vi "Create Plot Object.vi"(6 "Control Ref Queue":T1, 7 "Actual Transform In":T2, 8 "error in (no error)":errorcluster, 9 "Multiplot Representation In":T4, 10 "3D Mesh.lvclass in":refnum<class "3D Mesh.lvclass">, 11 "Plot Object In":refnum<vi>) -> (0 "error out":errorcluster, 1 "Multiplot Representation Out":T4, 2 "3D Mesh.lvclass out":refnum<class "3D Mesh.lvclass">, 3 "Plot Object Out":refnum<vi>, 5 "Actual Transform Out":T2)   [LabVIEW 2020, in "3D Mesh.lvclass"]
uses:
  <vilib>/Math Plots/3D Math Plots/3D Mesh/3D Mesh/3D Mesh.lvclass
  <vilib>/Math Plots/3D Math Plots/3D Plot/3D Plot/Typedef/Multiplot Representation.ctl
  <vilib>/Math Plots/3D Math Plots/3D Plot/3D Plot/Typedef/Plot Representation.ctl
  <vilib>/Math Plots/3D Math Plots/3D Plot/3D Plot/Typedef/Range Clusters.ctl
  <vilib>/Math Plots/3D Math Plots/3D Plot/3D Plot/Typedef/Mesh Data.ctl
  <vilib>/Math Plots/3D Math Plots/3D Plot/3D Plot/Typedef/Actual Transform.ctl
  <vilib>/Math Plots/3D Math Plots/3D Plot/Action String/3DMathPlot Ctrl Act Queue.ctl
  <vilib>/Math Plots/3D Math Plots/3D Plot/Action String/3DMathPlot Ctrl Act Cluster.ctl
  <vilib>/Math Plots/3D Math Plots/3D Plot/Action String/3DMathPlot State Class.ctl
  <vilib>/Math Plots/3D Math Plots/3D Mesh/3D Mesh/3D Mesh.lvclass/3D Mesh.ctl
  <vilib>/Math Plots/3D Math Plots/3D Plot/3D Plot/3D Plot.lvclass
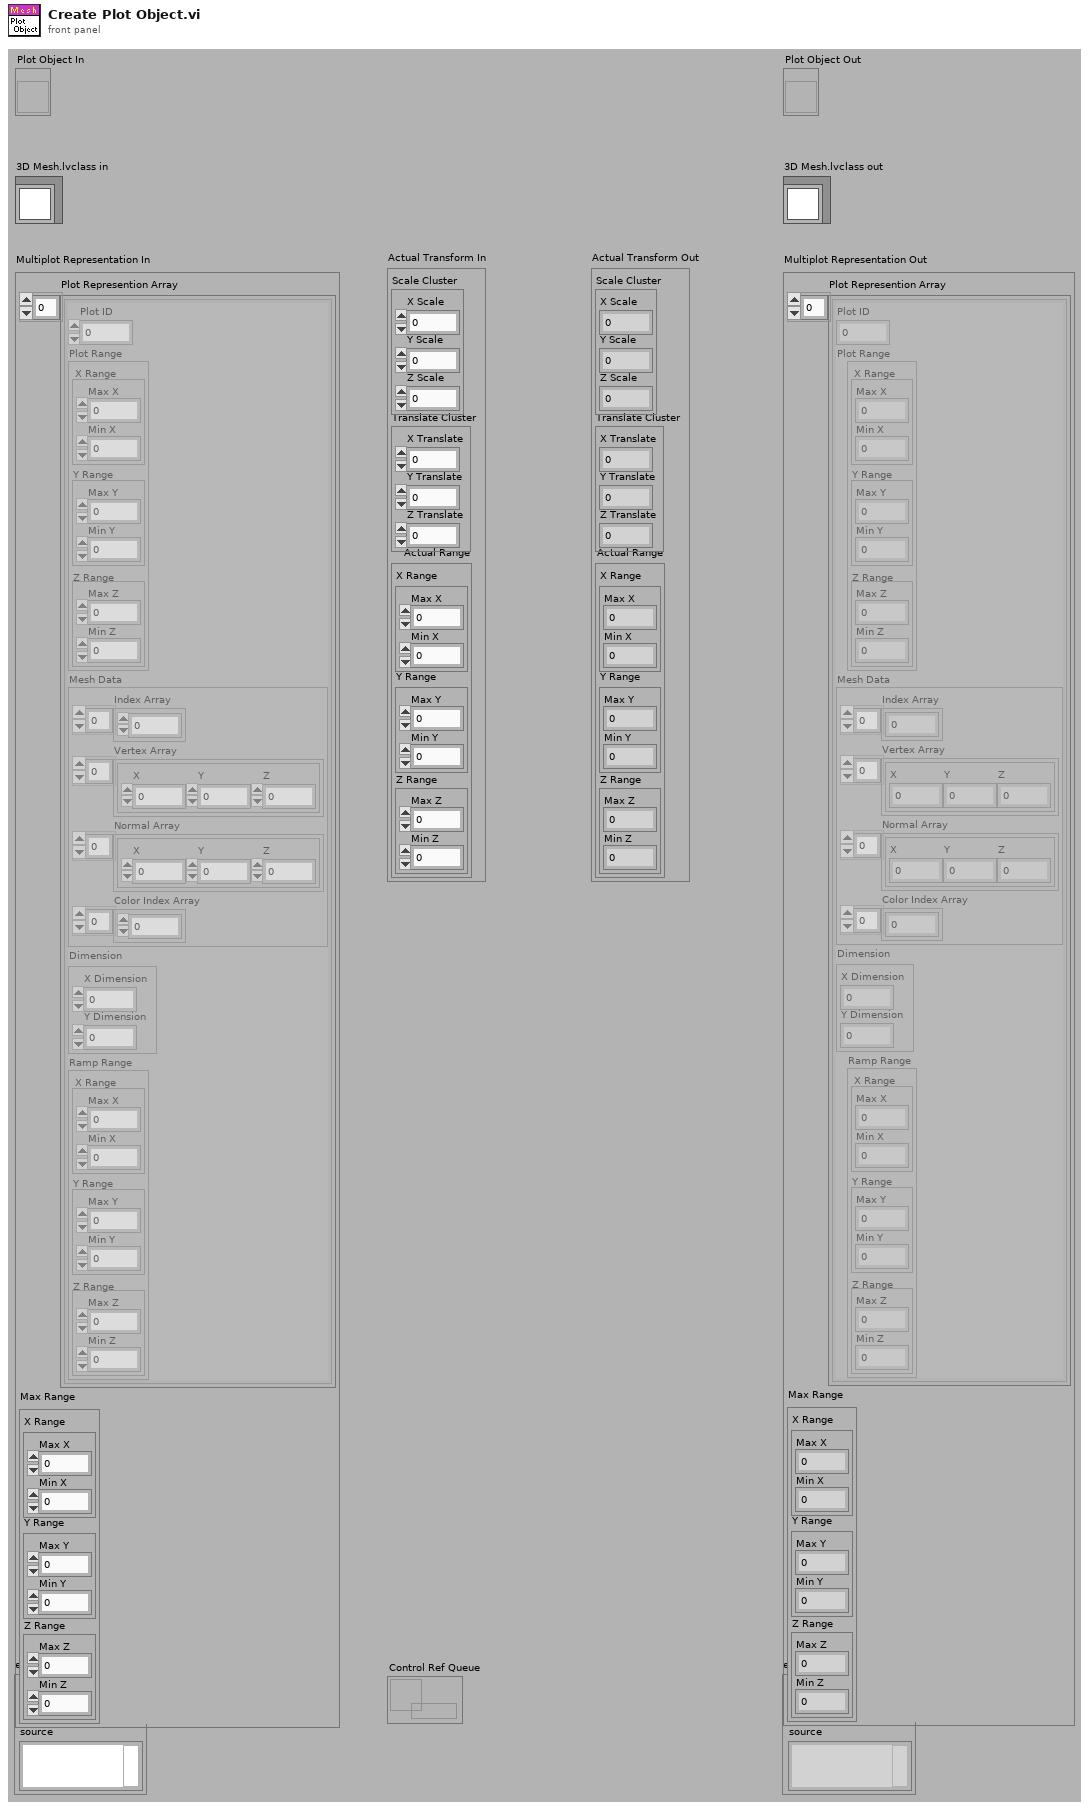
[diagram p1: front panel]
types:
  T1 = typedef "3DMathPlot Ctrl Act Queue.ctl" = refnum<queue>
  T2 = typedef "3D Plot.lvclass/Actual Transform.ctl" = cluster{"Scale Cluster":cluster{"X Scale":sgl, "Y Scale":sgl, "Z Scale":sgl}, "Translate Cluster":cluster{"X Translate":sgl, "Y Translate":sgl, "Z Translate":sgl}, "Actual Range":T3}
  T3 = typedef "3D Plot.lvclass/Range Clusters.ctl" = cluster{"X Range":cluster{"Max X":sgl, "Min X":sgl}, "Y Range":cluster{"Max Y":sgl, "Min Y":sgl}, "Z Range":cluster{"Max Z":sgl, "Min Z":sgl}}
  T4 = typedef "3D Plot.lvclass/Multiplot Representation.ctl" = cluster{"Plot Represention Array":T5[], "Max Range":T3}
  T5 = typedef "3D Plot.lvclass/Plot Representation.ctl" = cluster{"Plot ID":i32, "Plot Range":T3, "Mesh Data":T6, "Dimension":cluster{"X Dimension":i32, "Y Dimension":i32}, "Ramp Range":T3}
  T6 = typedef "3D Plot.lvclass/Mesh Data.ctl" = cluster{"Index Array":u32[], "Vertex Array":cluster{"X":sgl, "Y":sgl, "Z":sgl}[], "Normal Array":cluster{"X":sgl, "Y":sgl, "Z":sgl}[], "Color Index Array":i32[]}
  T7 = typedef "3D Mesh.lvclass/3D Mesh Propery Array.ctl" = T8[]
  T8 = typedef "3D Mesh.lvclass/3D Mesh Property.ctl" = cluster{"General Property":cluster{"Plot Name":string, "Coordinate System":enum16{"Cartesian", "Cylindrical", "Spherical"}, "Opacity":sgl}, "Projection Property":cluster{"Draw XY":bool, "Draw YZ":bool, "Draw XZ":bool}, "Plot Property":cluster{"Surface Color":u32, "Line Style":T9, "Line Width":sgl, "Color Ramp Cluster":T10, "Antialiasing":bool}, "Mesh Property":cluster{"Mesh Mode":enum16{"Lines", "Hidden Lines", "With Zero Plane"}}}
  T9 = typedef "3D Plot.lvclass/Line Type.ctl" = enum16{"None", "Solid", "Dash", "Dot", "Dash Dot"}
  T10 = typedef "3D Plot.lvclass/Color Ramp Cluster.ctl" = cluster{"Color Ramp Style":enum16{"None", "Shaded", "Color spectrum", "Grey scale", "Custom"}, "Color Ramp Array":u32[], "Color Ramp Index":i32[], "Interpolate?":bool, "Logarithm?":bool}
  T11 = enum16{"Points", "Lines", "Line Strip", "Line Loop", "Triangles", "Triangle Strip", "Triangle Fan", "Quads", "Quad Strip", "Polygon"}
  T12 = cluster{"Draw XY":bool, "Draw YZ":bool, "Draw XZ":bool}
  T13 = enum16{"Lines", "Hidden Lines", "With Zero Plane"}
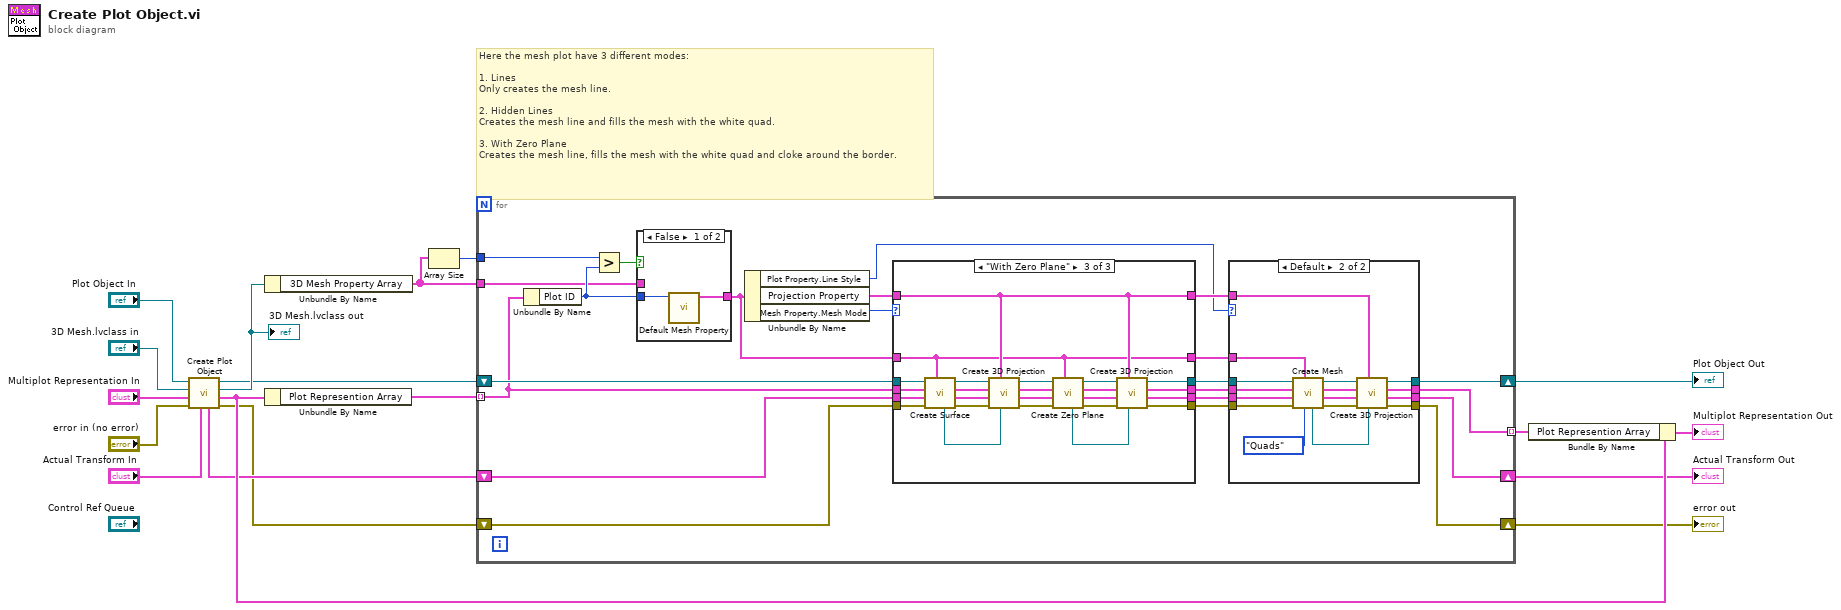
[diagram p0: block diagram]
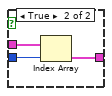
[diagram p2: hidden frame]
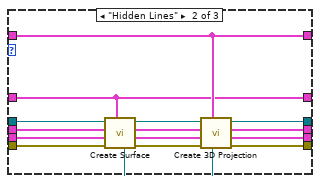
[diagram p5: hidden frame]
diagram:
  # "Here the mesh plot have 3 different modes:\n\n1. Lines\nOnly creates the mesh line.\n\n2. Hidden Lines\nCreates the mesh line and fills the mesh with the white quad.\n\n3. With Zero Plane\nCreates the mesh line, fills the mesh with the white quad and cloke around the border."
  n1 = call-parent "Create Plot Object.vi"("Actual Transform In"="Actual Transform In", "error in (no error)"="error in (no error)", "Multiplot Representation In"="Multiplot Representation In", "3D Plot.lvclass in"="3D Mesh.lvclass in", "Plot Object In"="Plot Object In") -> ("error out"=w6:errorcluster, "Multiplot Representation Out"=w12:T4, "3D Plot.lvclass out"=w5:refnum<class "3D Mesh.lvclass">, "Plot Object Out"=w4:refnum<vi>, "Actual Transform Out"=w9:T2)  [unwired: 1 in, 1 out]
  "3D Mesh.lvclass out" <- w5
  n2 = Unbundle By Name(w5) -> ("3D Mesh Property Array"=w2:T7)
  n3 = Unbundle By Name(w12) -> ("Plot Represention Array"=w18:T5[])
  n4 = Array Size(array=w2) -> (size(s)=w1:i32)
  n5 = for {
    shift-right: [w32] -> w7
    shift-left: w6 -> [w37]
    shift-right: [w30] -> w3
    shift-left: w4 -> [w40]
    shift-right: [w31] -> w8
    shift-left: w9 -> [w38]
    tunnel: w18 -> [w39] mode=indexing
    tunnel: [w27] -> w17 mode=indexing
    tunnel: w2 -> [w20]
    tunnel: w1 -> [w22]
    n6 = Unbundle By Name(w39) -> ("Plot ID"=w21:i32)
    n7 = Greater?(x=w22, y=w21) -> (0:w23:bool)
    n8 = case shown="False" w23 {
      tunnel: w20 -> [_ w45]
      tunnel: [w41 w44] -> w19
      tunnel: w21 -> [w42 w43]
      frame False {
        n9 = call <vilib>:"Default Mesh Property.vi"("Plot ID"=w42) -> ("Default Property"=w41:T8)  [unwired: 10 out]
      }
      frame True {
        n10 = Index Array(array=w45, index=w43) -> (element=w44:T8)
      }
    }
    n11 = Unbundle By Name(w19) -> ("Plot Property.Line Style"=w25:T9, "Projection Property"=w29:T12, "Mesh Property.Mesh Mode"=w24:T13)
    n12 = case shown="\"With Zero Plane\"" w24 {
      tunnel: [w70 w84 w106] -> w36
      tunnel: [w68 w83 w105] -> w34
      tunnel: [w69 w79 w90] -> w35
      tunnel: [w67 w78 w104] -> w33
      tunnel: w37 -> [w67 w76 w97]
      tunnel: w38 -> [w68 w75 w98]
      tunnel: w39 -> [w69 w74 w99]
      tunnel: w40 -> [w70 w73 w100]
      tunnel: w29 -> [w66 w72 w86]
      tunnel: w19 -> [w65 w71 w85]
      tunnel: [w66 w72 w86] -> w28
      tunnel: [w65 w71 w85] -> w26
      frame "Lines", Default {
      }
      frame "Hidden Lines" {
        n13 = call <vilib>:"Create Surface.vi"("3D Mesh Property"=w71, "error in (no error)"=w76, "Actual Transform In"=w75, "Plot Representation In"=w74, "Plot Object In"=w73) -> ("error out"=w82:errorcluster, "Actual Transform Out"=w80:T2, "Plot Representation Out"=w79:T5, "Plot Object Out"=w81:refnum<vi>, "Mesh Object Out"=w77:refnum<vi>)  [unwired: 2 in]
        n14 = call <vilib>:"Create 3D Projection.vi"("Sub Object In"=w77, "Projection Property"=w72, "error in (no error)"=w82, "Actual Transform In"=w80, "Plot Object In"=w81) -> ("error out"=w78:errorcluster, "Actual Transform Out"=w83:T2, "Plot Object Out"=w84:refnum<vi>)  [unwired: 1 in, 3 out]
      }
      frame "With Zero Plane" {
        n15 = call <vilib>:"Create Surface.vi"("3D Mesh Property"=w85, "error in (no error)"=w97, "Actual Transform In"=w98, "Plot Representation In"=w99, "Plot Object In"=w100) -> ("error out"=w96:errorcluster, "Actual Transform Out"=w95:T2, "Plot Representation Out"=w94:T5, "Plot Object Out"=w93:refnum<vi>, "Mesh Object Out"=w92:refnum<vi>)  [unwired: 2 in]
        n16 = call <vilib>:"Create 3D Projection.vi"("Sub Object In"=w92, "Projection Property"=w86, "error in (no error)"=w96, "Actual Transform In"=w95, "Plot Object In"=w93) -> ("error out"=w101:errorcluster, "Actual Transform Out"=w102:T2, "Plot Object Out"=w103:refnum<vi>)  [unwired: 1 in, 3 out]
        n17 = call <vilib>:"Create Zero Plane.vi"("3D Mesh Property"=w85, "error in (no error)"=w101, "Actual Transform In"=w102, "Plot Representation In"=w94, "Plot Object In"=w103) -> ("error out"=w89:errorcluster, "Actual Transform Out"=w88:T2, "Plot Representation Out"=w90:T5, "Plot Object Out"=w91:refnum<vi>, "Zero Plane Object Out"=w87:refnum<vi>)  [unwired: 2 in]
        n18 = call <vilib>:"Create 3D Projection.vi"("Sub Object In"=w87, "Projection Property"=w86, "error in (no error)"=w89, "Actual Transform In"=w88, "Plot Object In"=w91) -> ("error out"=w104:errorcluster, "Actual Transform Out"=w105:T2, "Plot Object Out"=w106:refnum<vi>)  [unwired: 1 in, 3 out]
      }
    }
    n19 = case shown="Default" w25 {
      tunnel: w36 -> [w49 w64]
      tunnel: w35 -> [w48 w63]
      tunnel: w34 -> [w47 w62]
      tunnel: w33 -> [w46 w61]
      tunnel: [w46 w55] -> w32
      tunnel: [w47 w54] -> w31
      tunnel: [w49 w53] -> w30
      tunnel: w28 -> [_ w52]
      tunnel: [w48 w51] -> w27
      tunnel: w26 -> [_ w50]
      frame "None" {
      }
      frame Default {
        n20 = call <vilib>:"Create Mesh.vi"("Draw Mode"=T11."Quads", "3D Mesh Property"=w50, "error in (no error)"=w61, "Actual Transform In"=w62, "Plot Representation In"=w63, "Plot Object In"=w64) -> ("error out"=w57:errorcluster, "Actual Transform Out"=w58:T2, "Plot Representation Out"=w51:T5, "Plot Object Out"=w59:refnum<vi>, "Mesh Object Out"=w56:refnum<vi>)  [unwired: 1 in]
        n21 = call <vilib>:"Create 3D Projection.vi"("Sub Object In"=w56, "Projection Property"=w52, "error in (no error)"=w57, "Actual Transform In"=w58, "Plot Object In"=w59) -> ("error out"=w55:errorcluster, "Actual Transform Out"=w54:T2, "Plot Object Out"=w53:refnum<vi>)  [unwired: 1 in, 3 out]
      }
    }
  }
  "error out" <- w7
  "Plot Object Out" <- w3
  "Actual Transform Out" <- w8
  n22 = Bundle By Name(cluster=w12, "Plot Represention Array"=w17) -> (→"Multiplot Representation Out":T4)
